vi "RT_Xdes_command_sharedvariable_example.vi"() -> ()   [LabVIEW 2019]
uses:
  <vilib>/Platform/TimedLoop/XDataNode/timing_clust.ctl
  <vilib>/Platform/TimedLoop/XDataNode/nitl_modes.ctl
  <vilib>/Platform/TimedLoop/XDataNode/wakeup.ctl
  <vilib>/platform/TimedLoop/XDataNode/XDataNode.xnode
  <vilib>/Platform/TimedLoop/XDataNode/XDNodeRunTimeDep.lvlib
panel:
  out "Data to save":dbl[](array[numeric])
  out "Xmeas Enc (mm)":dbl
  out "Xmeas IFO (mm)":dbl
  in  "stop":bool
  out "Xdes (mm)":dbl
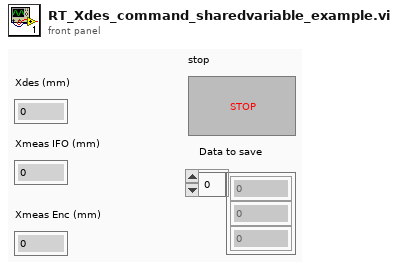
[diagram p1: front panel]
types:
  T1 = typedef "XDNodeRunTimeDep.lvlib/timing_clust.ctl" = cluster{"Expected End [f-1]":u64, "Actual End [f-1]":u64, "Finished Late? [f-1]":bool, "Expected End [i-1]":u64, "Actual End [i-1]":u64, "Finished Late? [i-1]":bool, "Expected Start [i]":u64, "Actual Start [i]":u64, "Expected Start [f]":u64, "Actual Start [f]":u64, "Source Name":string, "Structure Name":string, "Period":i64, "Deadline":i64, "Offset":i64, "Start":i64, "Priority":i32, "Timeout":i32, "Mode":T2, "Wakeup Reason":T3, "Error":errorcluster, "Source Type":string, "Secondary Source Type":string, "Global End Time":u64, "Global Start Time":u64, "Frame Duration":u64, "Iteration Duration":u64, "Assigned CPU":i32, "I/O Scan Engine Mode":u32}
  T2 = typedef "XDNodeRunTimeDep.lvlib/nitl_modes.ctl" = enum32{"No Change", "Process missed periods, maintain original phase", "Discard missed periods, maintain original phase", "Process missed periods, ignore original phase", "Discard missed periods, ignore original phase"}
  T3 = typedef "XDNodeRunTimeDep.lvlib/wakeup.ctl" = enum32{"Normal", "Aborted", "Asynchronous wakeup", "Timing source error", "Timed loop error", "Timeout"}
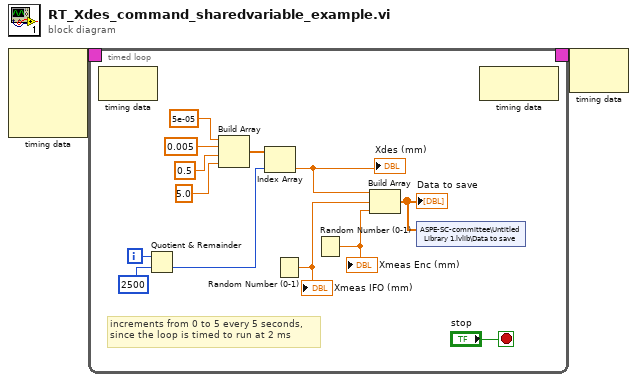
[diagram p0: block diagram]
diagram:
  n1 = node-c288() -> (w2:T1)  [unwired: 4 in]
  n2 = timed-loop {
    timing: w2 -> [_]
    timing-out: [_] -> w1
    i -> [w15]
    stop <- "stop" stop-if-true
    # "increments from 0 to 5 every 5 seconds,\nsince the loop is timed to run at 2 ms"
    n3 = node-c288() -> ()  [unwired: 1 in, 1 out]
    n4 = Quotient & Remainder(x=w15, y=2500) -> (floor(x/y)=w8:i32)  [unwired: 1 out]
    n5 = Build Array(5e-05 ("element"), 0.005 ("element"), 0.5 ("element"), 5.0 ("element")) -> (w9:dbl[])
    n6 = Index Array(array=w9, index=w8) -> (element=w6:dbl)
    "Xdes (mm)" <- w6
    n7 = Random Number (0-1)() -> (number: 0 to 1=w5:dbl)
    "Xmeas IFO (mm)" <- w5
    n8 = Random Number (0-1)() -> (number: 0 to 1=w4:dbl)
    "Xmeas Enc (mm)" <- w4
    n9 = Build Array(w6, w5, w4) -> (w3:dbl[])
    "Data to save" <- w3
    n10 = shared-variable "ASPE-SC-committee\\Untitled Library 1.lvlib\\Data to save"(w3) -> ()  [unwired: 1 in, 1 out]
    n11 = node-c288() -> ()  [unwired: 1 in, 1 out]
  }
  n12 = node-c288(w1) -> ()  [unwired: 1 out]
